vi "Point or Line Color List.vi"(2 "Color List":refnum<vi>) -> (7 "Point (T)/ Line (F)":bool)   [LabVIEW 2021, in "Graphs.lvlib"]
uses:
  Graphs.lvlib
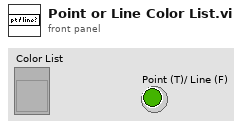
[diagram p1: front panel]
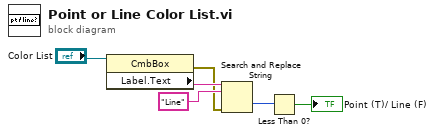
[diagram p0: block diagram]
diagram:
  n1 = property class="CmbBox"(reference="Color List") -> (error out=w3:errorcluster, "Label.Text"=w5:string)  [unwired: 1 in, 1 out]
  n2 = Search and Replace String(input string=w5, search string="Line", error in=w3) -> (offset past replacement=w2:i32)  [unwired: 5 in, 3 out]
  n3 = Less Than 0?(x=w2) -> (x < 0?=→"Point (T)/ Line (F)":bool)
